vi "Stop Event.vi"(2 "Input":refnum<user-event>, 3 "Action":T1) -> (0 "Output":refnum<user-event>)   [LabVIEW 2013]
uses:
  Functional Globals/Action.ctl
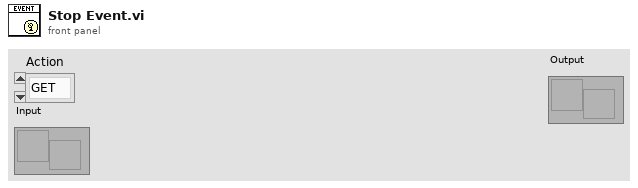
[diagram p1: front panel]
types:
  T1 = typedef "Action.ctl" = enum16{"GET", "PUT", "DELETE"}
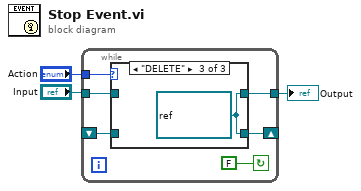
[diagram p0: block diagram]
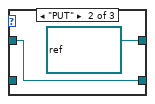
[diagram p3: hidden frame]
diagram:
  n1 = while {
    shift-right: [w7] -> _
    shift-left: _ -> [w6]
    tunnel: "Action" -> [w8]
    tunnel: "Input" -> [w5]
    tunnel: [w4] -> w1
    stop <- FALSE continue-if-true
    n2 = case shown="\"DELETE\"" w8 {
      tunnel: [w10 w12 w13] -> w7
      tunnel: w6 -> [w10 _ _]
      tunnel: w5 -> [_ w12 _]
      tunnel: [w10 refnum<user-event> refnum ("Input") w13] -> w4
      frame "GET", Default {
      }
      frame "PUT" {
      }
      frame "DELETE" {
        w13 = refnum<user-event> refnum ("Input")
      }
    }
  }
  "Output" <- w1
